vi "SPI Get Num Channels.vi"(8 "error in (no error)":errorcluster) -> (0 "error out":errorcluster, 3 "numChannels":u32)   [LabVIEW 2018, in "libMPSSE-SPI.lvlib"]
doc: "FTDI_API FT_STATUS SPI_GetNumChannels(uint32 *numChannels);"
uses:
  libMPSSE-SPI.lvlib
  dll/libMPSSE.dll
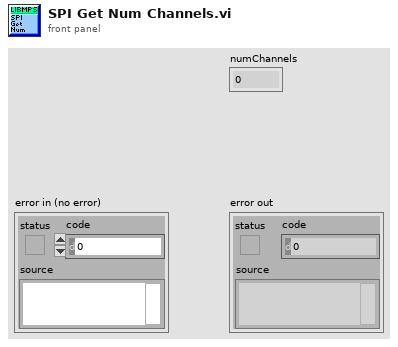
[diagram p1: front panel]
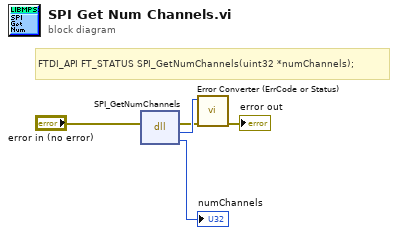
[diagram p0: block diagram]
diagram:
  # "FTDI_API FT_STATUS SPI_GetNumChannels(uint32 *numChannels);"
  n1 = dll-call lib="D:/LABVIEW/Examples - 32bit/FTDI/libMPSSE-SPI-LabVIEW-master/dll/libMPSSE.*" fn="SPI_GetNumChannels"(error in="error in (no error)") -> (error out=w2:errorcluster, w5:u32, "numChannels"=→"numChannels":u32)  [unwired: 3 in, 1 out]
  n2 = call "Error Converter (ErrCode or Status).vi"("error in (no error)"=w2, "error code"=w5) -> ("error out"=→"error out":errorcluster)  [unwired: 9 in]
